vi "Process.vi"(8 "error in":errorcluster, 11 "Logger":refnum<class "Logger.PGSQL.lvclass">) -> (0 "error out":errorcluster, 3 "Logger out":refnum<class "Logger.PGSQL.lvclass">)   [LabVIEW 2019, in "Logger.PGSQL.lvclass"]
doc: "---------------------------------------------------------------\nJKI State Machine Objects™\nhttp://jki.net/state-machine-objects/\nCopyright (C) 2005-2015, JKI <info@jki.net>\nALL RIGHTS RESERVED"
uses:
  Logger.PGSQL.lvclass
  C:/Program Files (x86)/National Instruments/LabVIEW 2019/vi.lib/JKI/JKI SMO/SMO/SMO.lvclass
  C:/Program Files (x86)/National Instruments/LabVIEW 2019/user.lib/LevyLab/Logger/Logger.lvclass
  <userlib>/LevyLab/LV-Data/LV-Data.PG/LV-Data.PGSQL.lvclass
  <vilib>/JKI/JKI SMO/SMO/SMO.lvclass/SMO.ctl
  <vilib>/JKI/JKI SMO/SMO/Private/ReftoDVR--SMO.vi
  <userlib>/LevyLab/LV-Data/LV-Data.PG/API/Write Variable (one-row).vi
  <userlib>/LevyLab/LV-Data/LV-Data.PG/API/Read Variable (string).vi
  <userlib>/LevyLab/Logger/Logger.lvclass
  <vilib>/JKI/JKI SMO/SMO/SMO.lvclass
panel:
  out "State History":string
  out "Status":string
  out "Data":variant
  out "Address(es)":string
  # "DB Logger"
  # "For instructions on how to use the JKI State Machine Objects, examples and video tutorials, visit:\nhttp://jki.net/state-machine-objects/\n\nJKI State Machine Objects™\nhttp://jki.net/state-machine-objects/\nCopyright (C) 2005-2015, JKI <info@jki.net>\nALL RIGHTS RESERVED"
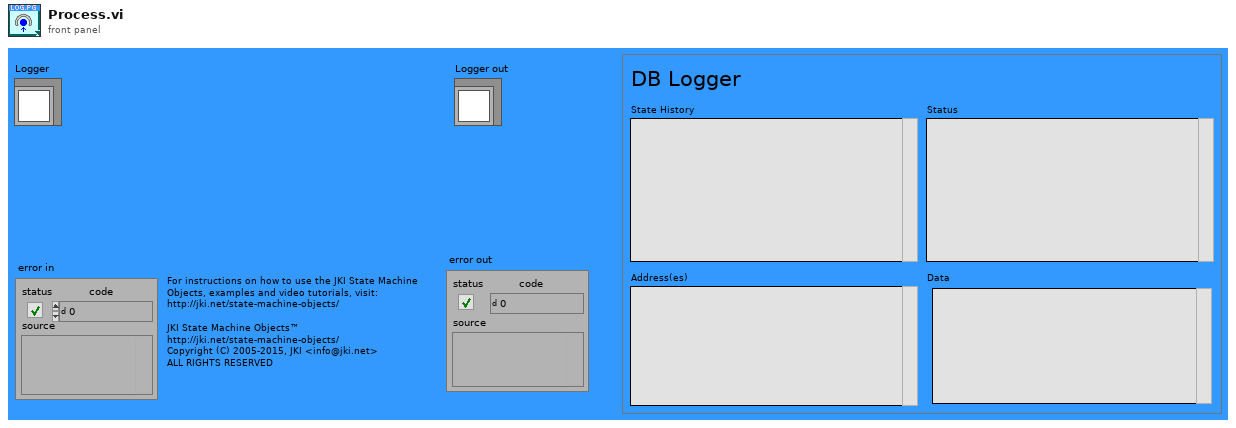
[diagram p1: front panel]
types:
  T1 = enum32{"invalid app kind", "Development System", "Run Time System", "Student Edition", "Embedded LabVIEW", "Evaluation", "Custom"}
  T2 = enum32{"Invalid", "Standard", "Closed", "Hidden", "Minimized", "Maximized"}
  T3 = enum32{"Bad", "Idle", "Run top level", "Running"}
  T4 = cluster{"Core":cluster{"Current VI Reference":refnum<vi>, "Close Panel on Exit?":bool, "Last Error":cluster{"error":errorcluster, "previous state":string, "remaining states":string}, "Shutdown?":bool}, "SelfRef":refnum<class "Logger.PGSQL.lvclass">, "Data.PGSQL":refnum<class "LV-Data.PGSQL.lvclass">, "variable address":string, "data in":variant, "data out":variant, "Debug Mode?":bool, "Time":timestamp}
  T5 = cluster{"Current VI Reference":refnum<vi>, "Close Panel on Exit?":bool, "Last Error":cluster{"error":errorcluster, "previous state":string, "remaining states":string}, "Shutdown?":bool}
  T6 = typedef "SMO.lvclass/Protected Events.ctl" = cluster{"StopProcesses":refnum<user-event>, "AbortProcesses":refnum<user-event>, "Config Changed":refnum<user-event>, "Dependency":refnum<user-event>}
  T7 = typedef "Logger.PGSQL.lvclass/PrivateEvents--Cluster.ctl" = cluster{"Set Address":refnum<user-event>, "Write Variable":refnum<user-event>, "Read Variable":refnum<user-event>}
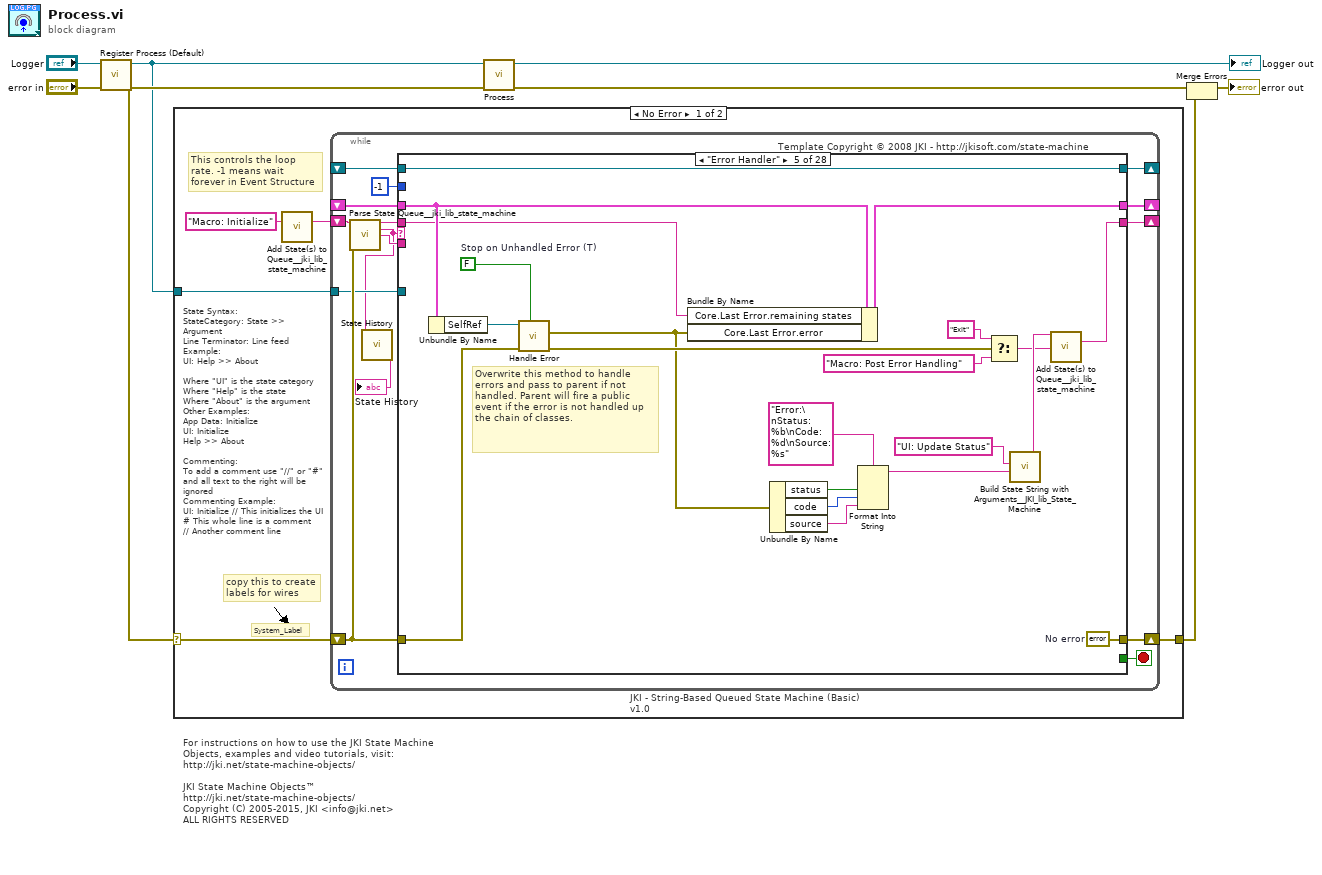
[diagram p0: block diagram]
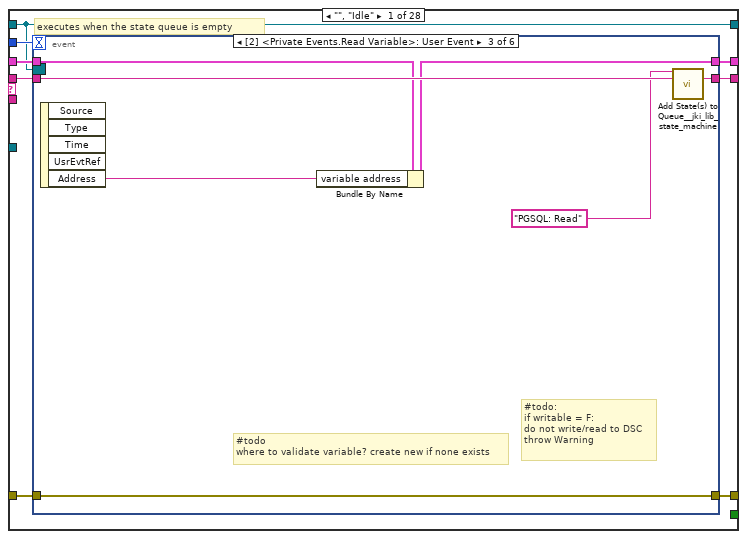
[diagram p2: hidden frame]
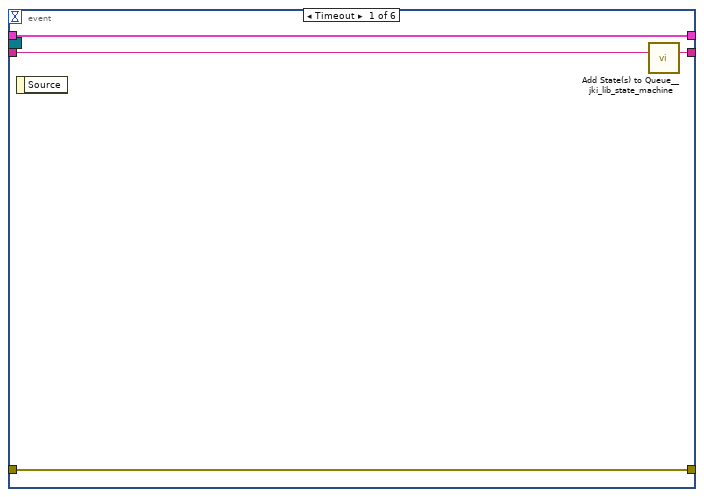
[diagram p3: hidden frame]
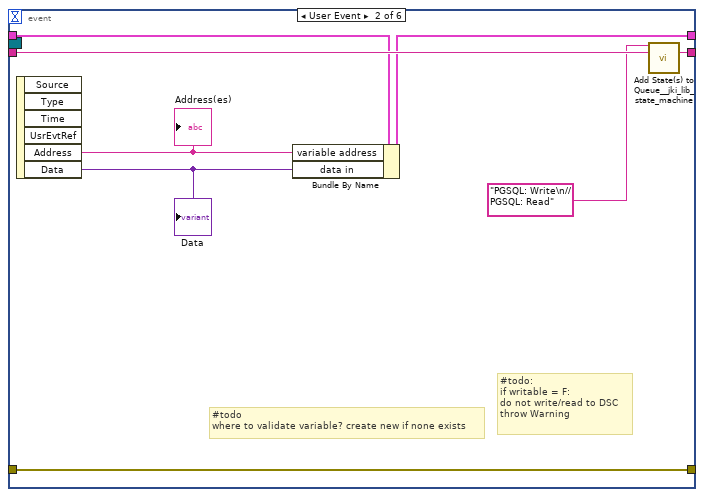
[diagram p4: hidden frame]
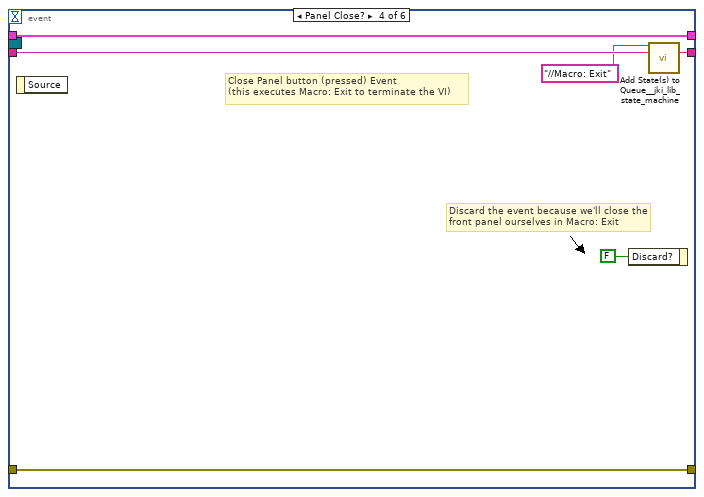
[diagram p5: hidden frame]
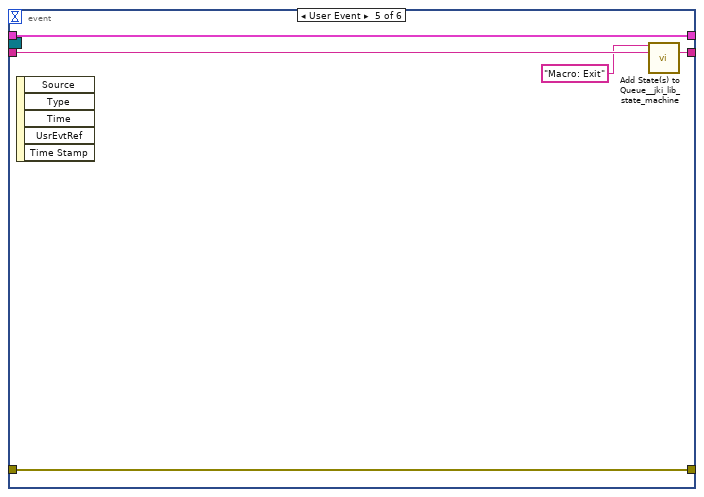
[diagram p6: hidden frame]
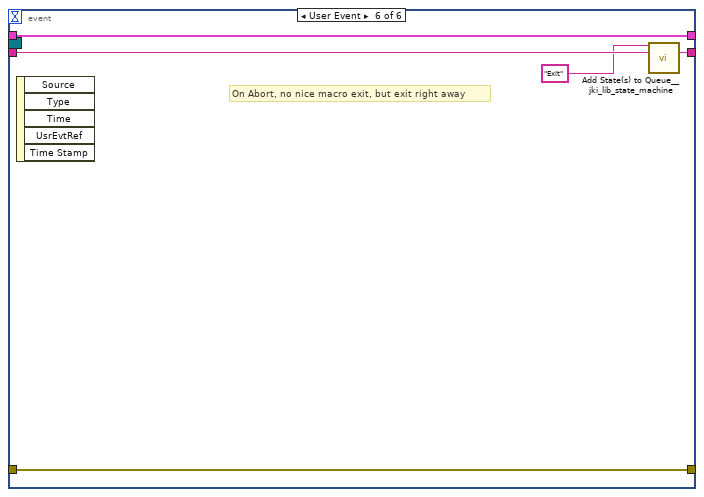
[diagram p7: hidden frame]
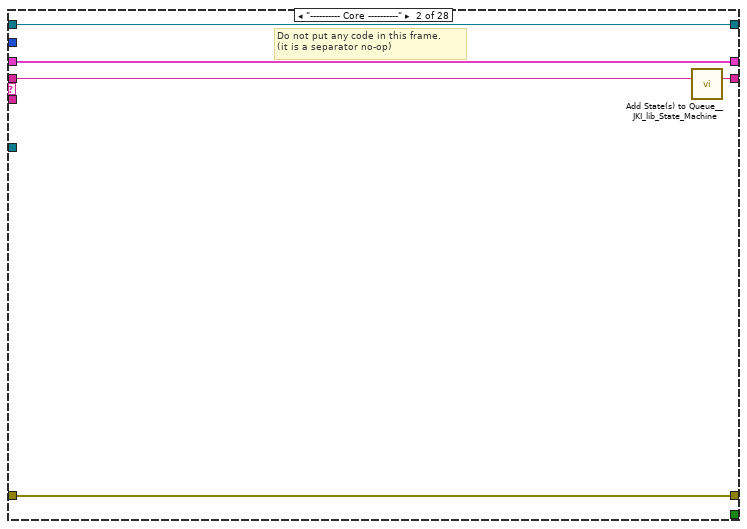
[diagram p8: hidden frame]
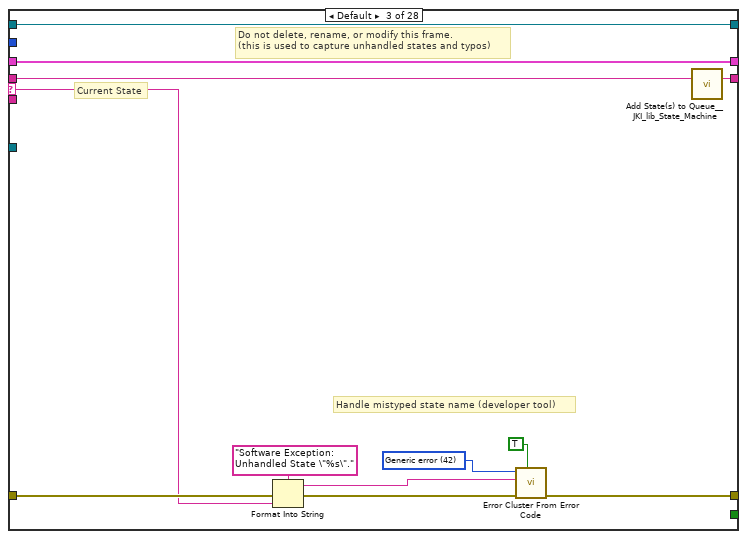
[diagram p9: hidden frame]
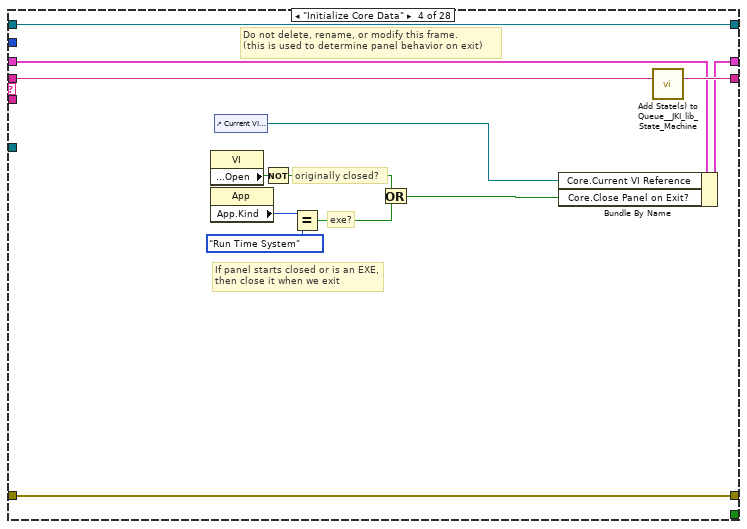
[diagram p10: hidden frame]
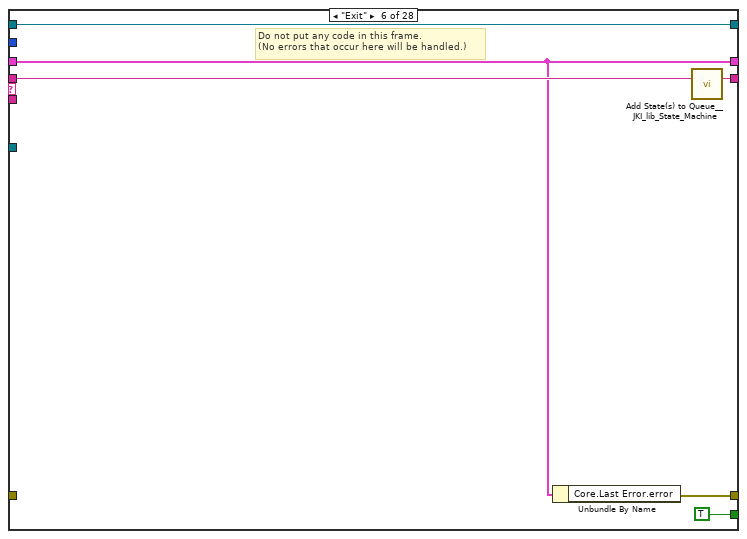
[diagram p11: hidden frame]
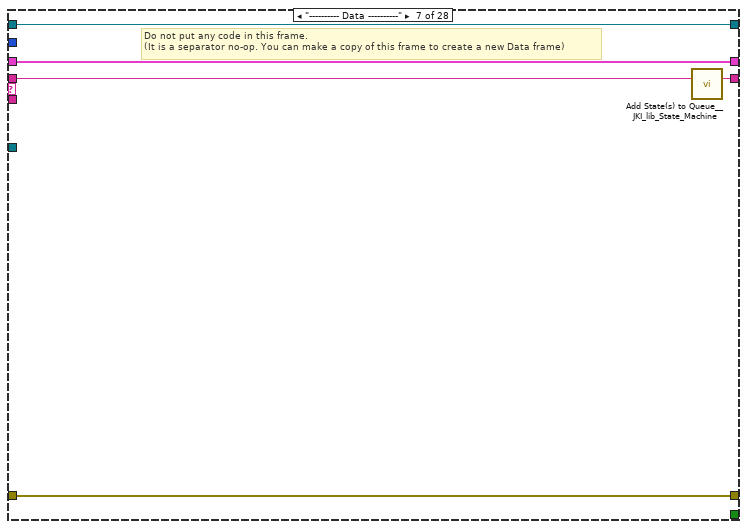
[diagram p12: hidden frame]
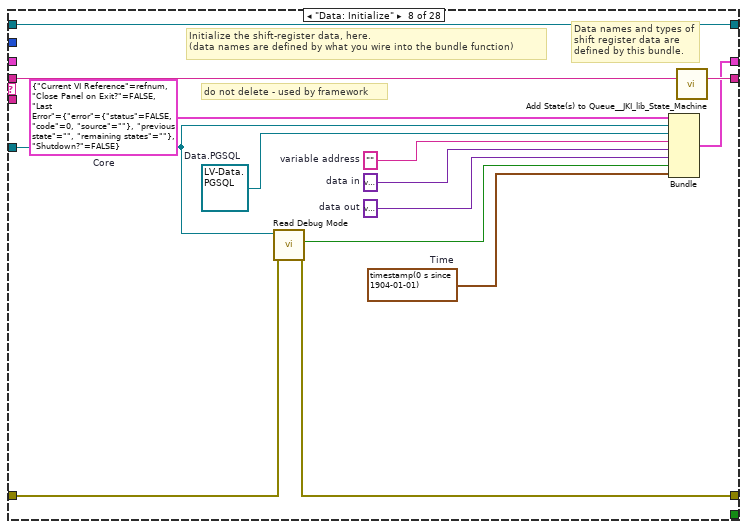
[diagram p13: hidden frame]
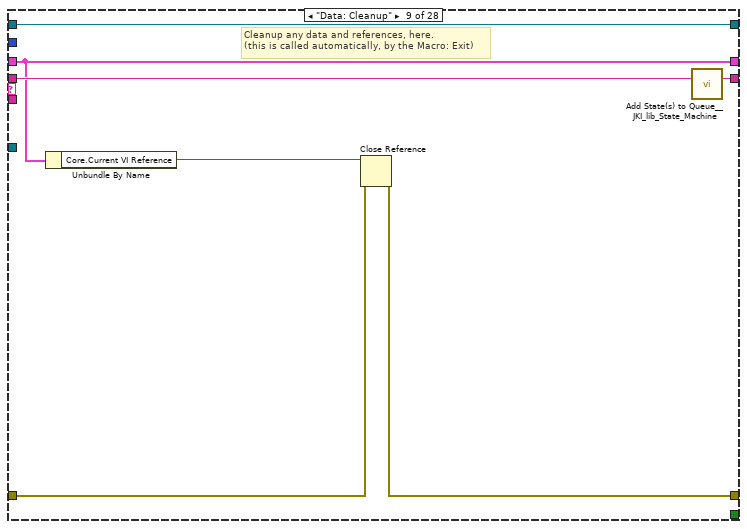
[diagram p14: hidden frame]
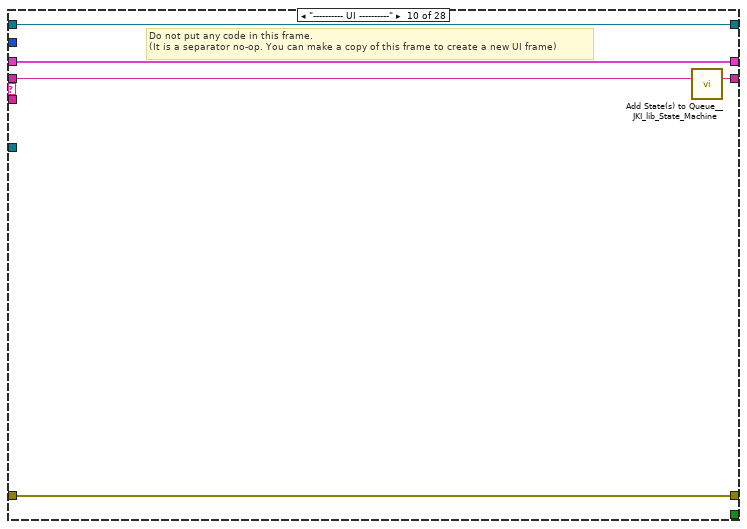
[diagram p15: hidden frame]
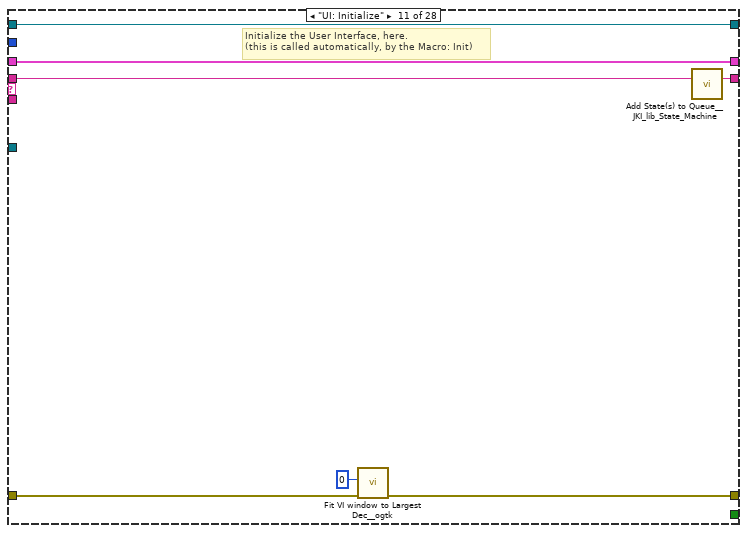
[diagram p16: hidden frame]
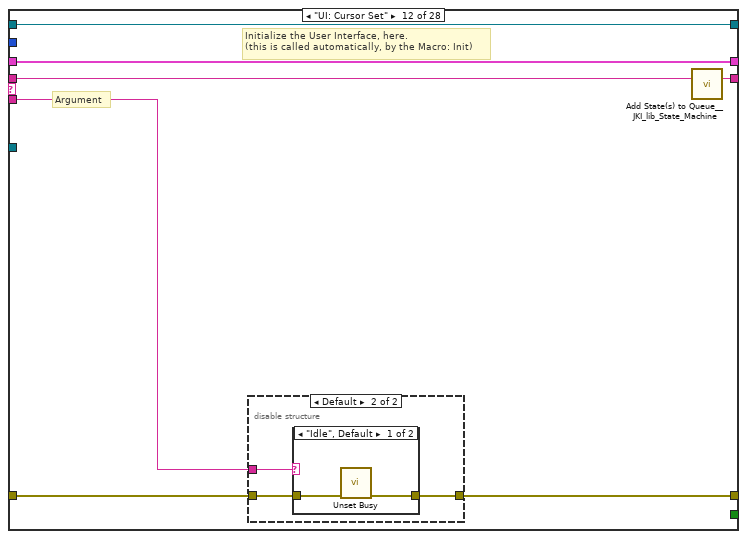
[diagram p17: hidden frame]
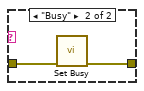
[diagram p19: hidden frame]
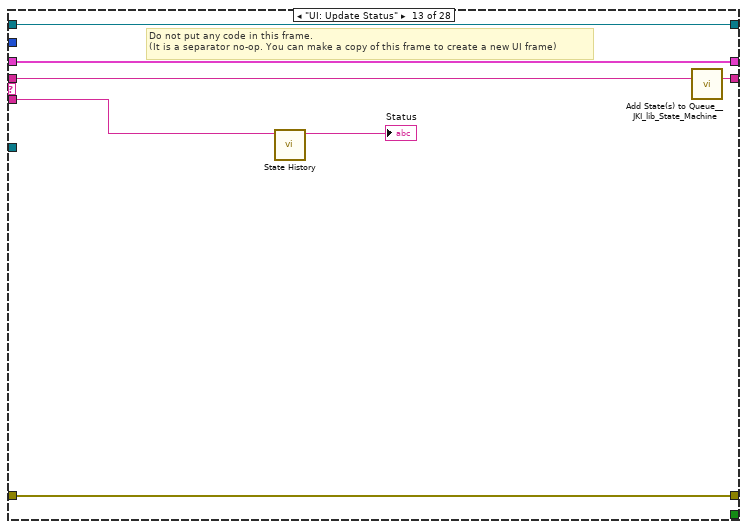
[diagram p20: hidden frame]
diagram:
  # "For instructions on how to use the JKI State Machine Objects, examples and video tutorials, visit:\nhttp://jki.net/state-machine-objects/\n\nJKI State Machine Objects™\nhttp://jki.net/state-machine-objects/\nCopyright (C) 2005-2015, JKI <info@jki.net>\nALL RIGHTS RESERVED"
  n1 = call <vilib>:"Register Process (Default).vi"("error in (no error)"="error in", "SMO"="Logger") -> ("error out"=w5:errorcluster, "SelfRef"=w4:refnum<class "Logger.PGSQL.lvclass">)  [unwired: 8 in]
  n2 = case shown="No Error" w5 {
    selector: w5 -> [w10 w412]
    tunnel: w4 -> [w11 _]
    tunnel: [w9 w412] -> w2
    frame No Error {
      # "State Syntax:\nStateCategory: State >> Argument\nLine Terminator: Line feed\nExample:\nUI: Help >> About\n\nWhere \"UI\" is the state category\nWhere \"Help\" is the state\nWhere \"About\" is the argument\nOther Examples:\nApp Data: Initialize\nUI: Initialize\nHelp >> About\n\nCommenting:\nTo add a comment use \"//\" or \"#\" and all text to the right will be ignored\nCommenting Example:\nUI: Initialize // This initializes the UI\n# This whole line is a comment\n// Another comment line"
      # "copy this to create labels for wires"
      # "This controls the loop rate. -1 means wait forever in Event Structure"
      # "System_Label"
      n3 = call <vilib>:"Add State(s) to Queue__jki_lib_state_machine.vi"("State(s) in (\"\")"="Macro: Initialize") -> ("States Out"=w13:string)  [unwired: 14 in]
      n4 = while "JKI - String-Based Queued State Machine (Basic) v1.0" {
        shift-right: [w22] -> _
        shift-left: _ -> [w21]
        shift-right: [w25] -> w9
        shift-left: w10 -> [w19]
        shift-right: [w24] -> _
        shift-left: w13 -> [w26]
        tunnel: w11 -> [w18]
        shift-right: [w17] -> _
        shift-left: _ -> [w16]
        stop <- w23 stop-if-true
        # "Template Copyright © 2008 JKI - http://jkisoft.com/state-machine"
        n5 = call <vilib>:"Parse State Queue__jki_lib_state_machine.vi"("State Queue"=w26, "Error In (no error)"=w19) -> ("Remaining States"=w28:string, "Current State"=w14:string, "Arguments"=w27:string)  [unwired: 11 in]
        n6 = call <userlib>:"State History.vi"("Current State"=w14) -> ("History"=→"State History":string)  [unwired: 10 in]
        n7 = case shown="\"Error Handler\"" w14 {
          selector: w14 -> [_ _ w78 _ _ _ _ _ _ _ _ _ _ _ _ _ _ _ _ _ _ _ _ _ _ _ _ _]
          tunnel: w28 -> [w36 w76 w82 w101 w108 w128 w133 w147 w154 w159 w166 w173 w188 w196 w228 w251 w263 w286 w291 w302 w307 w320 w326 w331 w340 w364 w394 w411]
          tunnel: w27 -> [_ _ _ _ _ _ _ _ _ _ _ w167 w182 w190 _ _ _ _ _ _ _ _ _ _ _ _ _ _]
          tunnel: w21 -> [w34 w73 w80 w92 w118 w124 w130 _ w149 w156 w164 w171 w185 w192 w225 w236 w253 w278 w288 w299 w304 w318 w324 w329 w332 w359 w387 w406]
          tunnel: [w33 w74 w84 w98 w119 w123 w131 w140 w150 w157 w162 w168 w186 w193 w226 w232 w261 w284 w289 w293 w305 w313 w322 w327 w335 w361 w391 w403] -> w25
          tunnel: w19 -> [w32 w74 w83 w98 w120 _ w131 w134 w151 w157 w161 w169 w186 w194 w226 w231 w261 w284 w289 w294 w305 w314 w322 w327 w333 w356 w388 w404]
          tunnel: [w35 w75 w81 w100 w104 w127 w132 w146 w153 w158 w165 w172 w187 w195 w227 w250 w262 w285 w290 w301 w306 w319 w325 w330 w339 w363 w393 w410] -> w24
          tunnel: [_ _ _ _ _ TRUE _ _ _ _ _ _ _ _ _ _ _ _ _ _ _ _ _ _ _ _ _ _] -> w23
          tunnel: [w31 w73 w80 w99 w117 w124 w130 w145 w149 w156 w164 w171 w185 w192 w225 w236 w254 w278 w288 w299 w304 w318 w324 w329 w337 w358 w387 w405] -> w22
          tunnel: -1 ("Timeout") -> [w30 _ _ _ _ _ _ _ _ _ _ _ _ _ _ _ _ _ _ _ _ _ _ _ _ _ _ _]
          tunnel: w18 -> [_ _ _ _ _ _ _ w135 _ _ _ _ _ _ _ w230 _ _ _ _ _ _ _ _ _ _ _ _]
          tunnel: [w29 w72 w77 w89 w122 w125 w129 w144 w148 w155 w163 w170 w184 w189 w224 w249 w260 w279 w287 w300 w303 w317 w323 w328 w338 w362 w392 w409] -> w17
          tunnel: w16 -> [w29 w72 w77 w89 w122 w125 w129 w144 w148 w155 w163 w170 w184 w189 w224 w249 w260 w279 w287 w300 w303 _ w323 w328 w338 w362 w392 w409]
          frame "", "Idle" {
            # "executes when the state queue is empty"
            n8 = event shown="[2] <Private Events.Read Variable>: User Event" {
              selector: w29 -> [_ _ _ _ _ _]
              dyn-events: _ -> [_ _ _ _ _ _]
              timeout: w30 -> [_ _ _ _ _ _]
              tunnel: w36 -> [w40 w48 w55 w61 w66 w71]
              tunnel: [w39 w47 w54 w60 w65 w70] -> w35
              tunnel: w34 -> [w38 w45 w52 w58 w63 w68]
              tunnel: [w37 w46 w53 w59 w64 w69] -> w33
              tunnel: w32 -> [w37 w46 w53 w59 w64 w69]
              tunnel: [w38 w44 w51 w58 w63 w68] -> w31
              event Timeout {
                n9 = event-data() -> ()  [unwired: 1 in, 1 out]
                n10 = call <vilib>:"Add State(s) to Queue__jki_lib_state_machine.vi"("State(s) in (\"\")"=w40) -> ("States Out"=w39:string)  [unwired: 14 in]
              }
              event User Event {
                # "#todo:\nif writable = F:\ndo not write/read to DSC\nthrow Warning"
                # "#todo\nwhere to validate variable? create new if none exists"
                n11 = event-data() -> ("Address"=w41:string, "Data"=w42:variant)  [unwired: 1 in, 4 out]
                "Address(es)" <- w41
                "Data" <- w42
                n12 = Bundle By Name(cluster=w45, "variable address"=w41, "data in"=w42) -> (w44:T4)
                n13 = call <vilib>:"Add State(s) to Queue__jki_lib_state_machine.vi"("State(s) in Front (\"\")"="PGSQL: Write\n//PGSQL: Read" ("State(s) in Front (\"\")"), "State(s) in (\"\")"=w48) -> ("States Out"=w47:string)  [unwired: 13 in]
              }
              event User Event {
                # "#todo:\nif writable = F:\ndo not write/read to DSC\nthrow Warning"
                # "#todo\nwhere to validate variable? create new if none exists"
                n14 = event-data() -> ("Address"=w49:string)  [unwired: 1 in, 4 out]
                n15 = Bundle By Name(cluster=w52, "variable address"=w49) -> (w51:T4)
                n16 = call <vilib>:"Add State(s) to Queue__jki_lib_state_machine.vi"("State(s) in Front (\"\")"="PGSQL: Read" ("State(s) in Front (\"\")"), "State(s) in (\"\")"=w55) -> ("States Out"=w54:string)  [unwired: 13 in]
              }
              event Panel Close? {
                # "Discard the event because we'll close the front panel ourselves in Macro: Exit"
                # "Close Panel button (pressed) Event\n(this executes Macro: Exit to terminate the VI)"
                n17 = event-data() -> ()  [unwired: 1 in, 1 out]
                n18 = event-data("Discard?"=FALSE) -> ()  [unwired: 1 in, 1 out]
                n19 = call <vilib>:"Add State(s) to Queue__jki_lib_state_machine.vi"("State(s) in Front (\"\")"="//Macro: Exit", "State(s) in (\"\")"=w61) -> ("States Out"=w60:string)  [unwired: 13 in]
              }
              event User Event {
                n20 = event-data() -> ()  [unwired: 1 in, 5 out]
                n21 = call <vilib>:"Add State(s) to Queue__jki_lib_state_machine.vi"("State(s) in Front (\"\")"="Macro: Exit", "State(s) in (\"\")"=w66) -> ("States Out"=w65:string)  [unwired: 13 in]
              }
              event User Event {
                # "On Abort, no nice macro exit, but exit right away"
                n22 = event-data() -> ()  [unwired: 1 in, 5 out]
                n23 = call <vilib>:"Add State(s) to Queue__jki_lib_state_machine.vi"("State(s) in Front (\"\")"="Exit", "State(s) in (\"\")"=w71) -> ("States Out"=w70:string)  [unwired: 13 in]
              }
            }
          }
          frame "---------- Core ----------" {
            # "Do not put any code in this frame.\n(it is a separator no-op)"
            n24 = call <vilib>:"Add State(s) to Queue__JKI_lib_State_Machine.vi"("State(s) in (\"\")"=w76) -> ("States Out"=w75:string)  [unwired: 14 in]
          }
          frame Default {
            w87 = 42 items=["No error", "Argument error", "Memory is full", "Out of zone", "End of file", "File already open", "Generic file I/O error", "File not found", "File permission error", "Disk is full", "Duplicate path", "Too many files open", "System feature not enabled", "Resource file not found", "Cannot add resource", "Resource not found", "Image not found", "Image memory error", "Pen does not exist", "Config type invalid", "Config token not found", "Config parse error", "Config memory error", "Bad external code format", "Bad external code offset", "External code not present", "Null window", "Destroy window error", "Null menu", "Print aborted", "Bad print record", "Print driver error", "Windows error during printing", "Memory error during printing", "Print dialog error", "Generic print error", "Invalid device refnum", "Device not found", "Device parameter error", "Device unit error", "Cannot open device", "Device call aborted", "Generic error", "Cancelled by user", "Object ID too low", "Object ID too high", "Object not in heap", "Unknown heap", "Unknown object (invalid DefProc)", "Unknown object (DefProc not in table)", "Message out of range", "Invalid (null) method", "Unknown message", "Manager call not supported", "Bad address", "Network operation in progress", "Network operation timed out", "Connection is busy", "Network attribute not supported", "Network error", "Address in use", "System out of memory", "Connection aborted", "Connection refused", "Not connected", "Already connected", "Connection closed", "Initialization error (interapplication manager)", "Bad occurrence", "Wait on unbound occurrence handler", "Occurrence queue overflow", "Datalog type conflict", "Unused", "Unrecognized type (interapplication manager)", "Memory corrupt", "Failed to make temporary DLL", "Old CIN version", "Drag socket not found", "Failed to load drop-object", "Failed to register OLE object", "Failed to release OLE object", "Format specifier type mismatch", "Unknown format specifier", "Too few format specifiers", "Too many format specifiers", "Scan failed", "Newer CIN version", "Error converting to variant", "Runtime menu error", "Password tampered", "Variant attribute not found", "Incompatible variant data type", "Event data is not available", "Event Store is not present", "Occurrence is not found", "Event Queue is not created", "Event info is not available", "Refnum passed is NULL", "Error retrieving Class GUID", "Error retrieving CoClass GUID", "Error retrieving TypeLib GUID.", "Bad built application magic bytes.", "Specific driver is different from the specific driver associated with the Logical Name.", "There is no session opened to the class driver.", "Max Error", "MAX - Error with config objects", "MAX - Error loading configuration", "MAX - Group not supported"]
            # "Current State"
            # "Do not delete, rename, or modify this frame.\n(this is used to capture unhandled states and typos)"
            # "Handle mistyped state name (developer tool)"
            n25 = Format Into String(format string="Software Exception: Unhandled State \"%s\"." ("message"), error in=w83, w78) -> (resulting string=w86:string, error out=w85:errorcluster)  [unwired: 1 in]
            n26 = call <vilib>:"Error Cluster From Error Code.vi"("show call chain? (False)"=TRUE, "error in (no error)"=w85, "error message (\"\")"=w86, "error code (0)"=w87) -> ("error out"=w84:errorcluster)  [unwired: 5 in]
            n27 = call <vilib>:"Add State(s) to Queue__JKI_lib_State_Machine.vi"("State(s) in (\"\")"=w82) -> ("States Out"=w81:string)  [unwired: 14 in]
          }
          frame "Initialize Core Data" {
            # "Do not delete, rename, or modify this frame.\n(this is used to determine panel behavior on exit)"
            # "originally closed?"
            # "exe?"
            # "If panel starts closed or is an EXE, then close it when we exit"
            n28 = property class="VI"() -> ("Front Panel.Open"=w97:bool)  [unwired: 2 in, 2 out]
            n29 = property class="App"() -> ("App.Kind"=w96:T1)  [unwired: 2 in, 2 out]
            n30 = control-ref of="Current VI Reference"() -> (w90:refnum<vi>)
            n31 = Not(x=w97) -> (.not. x?=w94:bool)
            n32 = Equal?(x=w96, y=T1."Run Time System" ("Application:Kind")) -> (x = y?=w93:bool)
            n33 = Or(x=w94, y=w93) -> (x .or. y?=w91:bool)
            n34 = Bundle By Name(cluster=w92, "Core.Current VI Reference"=w90, "Core.Close Panel on Exit?"=w91) -> (w99:T4)
            n35 = call <vilib>:"Add State(s) to Queue__JKI_lib_State_Machine.vi"("State(s) in (\"\")"=w101) -> ("States Out"=w100:string)  [unwired: 14 in]
          }
          frame "Error Handler" {
            w114 = FALSE  # Stop on Unhandled Error (T)
            w119 = errorcluster {"status"=FALSE, "code"=0, "source"=""}  # No error
            # "Overwrite this method to handle errors and pass to parent if not handled. Parent will fire a public event if the error is not handled up the chain of classes."
            n36 = Unbundle By Name(w118) -> ("SelfRef"=w121:refnum<class "Logger.PGSQL.lvclass">)
            n37 = call-dynamic "Handle Error.vi"("Stop on Unhandled Error (T)"=w114, "error in"=w120, "SMO"=w121) -> ("handling error"=w115:errorcluster, "Unhandled error"=w113:errorcluster)  [unwired: 6 in, 1 out]
            n38 = Bundle By Name(cluster=w118, "Core.Last Error.remaining states"=w108, "Core.Last Error.error"=w113) -> (w117:T4)
            n39 = Unbundle By Name(w113) -> ("status"=w112:bool, "code"=w110:i32, "source"=w109:string)
            n40 = Format Into String(format string="Error:\nStatus: %b\nCode: %d\nSource: %s", w112, w110, w109) -> (resulting string=w103:string)  [unwired: 2 in, 1 out]
            n41 = Select(t="Exit", s=w115, f="Macro: Post Error Handling") -> (s? t:f=w105:string)
            n42 = call <vilib>:"Build State String with Arguments__JKI_lib_State_Machine.vi"("Arguments (\"\")"=w103, "State"="UI: Update Status") -> ("State with Arguments"=w106:string)  [unwired: 4 in]
            n43 = call <vilib>:"Add State(s) to Queue__jki_lib_state_machine.vi"("State(s) in Front (\"\")"=w106, "State(s) at Back (\"\")"=w105) -> ("States Out"=w104:string)  [unwired: 13 in]
          }
          frame "Exit" {
            # "Do not put any code in this frame.\n(No errors that occur here will be handled.)"
            n44 = Unbundle By Name(w124) -> ("Core.Last Error.error"=w123:errorcluster)
            n45 = call <vilib>:"Add State(s) to Queue__JKI_lib_State_Machine.vi"("State(s) in (\"\")"=w128) -> ("States Out"=w127:string)  [unwired: 14 in]
          }
          frame "---------- Data ----------" {
            # "Do not put any code in this frame.\n(It is a separator no-op. You can make a copy of this frame to create a new Data frame)"
            n46 = call <vilib>:"Add State(s) to Queue__JKI_lib_State_Machine.vi"("State(s) in (\"\")"=w133) -> ("States Out"=w132:string)  [unwired: 14 in]
          }
          frame "Data: Initialize" {
            w136 = timestamp(0 s since 1904-01-01)  # Time
            w137 = refnum<class "LV-Data.PGSQL.lvclass"> refnum  # Data.PGSQL
            w138 = variant  # data out
            w141 = variant  # data in
            w142 = ""  # variable address
            w143 = T5 {"Current VI Reference"=refnum, "Close Panel on Exit?"=FALSE, "Last Error"={"error"={"status"=FALSE, "code"=0, "source"=""}, "previous state"="", "remaining states"=""}, "Shutdown?"=FALSE}  # Core
            # "do not delete - used by framework"
            # "Data names and types of shift register data are defined by this bundle."
            # "Initialize the shift-register data, here.\n(data names are defined by what you wire into the bundle function)"
            n47 = call <userlib>:"Read Debug Mode.vi"("error in (no error)"=w134, "Logger in"=w135) -> ("error out"=w140:errorcluster, "Debug Mode?"=w139:bool)  [unwired: 7 in, 1 out]
            n48 = Bundle("Core"=w143, "SelfRef"=w135, "Data.PGSQL"=w137, "variable address"=w142, "data in"=w141, "data out"=w138, "Debug Mode?"=w139, "Time"=w136) -> (w145:T4)  [unwired: 1 in]
            n49 = call <vilib>:"Add State(s) to Queue__JKI_lib_State_Machine.vi"("State(s) in (\"\")"=w147) -> ("States Out"=w146:string)  [unwired: 14 in]
          }
          frame "Data: Cleanup" {
            # "Cleanup any data and references, here.\n(this is called automatically, by the Macro: Exit)"
            n50 = Unbundle By Name(w149) -> ("Core.Current VI Reference"=w152:refnum<vi>)
            n51 = Close Reference(reference=w152, error in (no error)=w151) -> (error out=w150:errorcluster)
            n52 = call <vilib>:"Add State(s) to Queue__JKI_lib_State_Machine.vi"("State(s) in (\"\")"=w154) -> ("States Out"=w153:string)  [unwired: 14 in]
          }
          frame "---------- UI ----------" {
            # "Do not put any code in this frame.\n(It is a separator no-op. You can make a copy of this frame to create a new UI frame)"
            n53 = call <vilib>:"Add State(s) to Queue__JKI_lib_State_Machine.vi"("State(s) in (\"\")"=w159) -> ("States Out"=w158:string)  [unwired: 14 in]
          }
          frame "UI: Initialize" {
            # "Initialize the User Interface, here.\n(this is called automatically, by the Macro: Init)"
            n54 = call <userlib>:"Fit VI window to Largest Dec__ogtk.vi"("error in (no error)"=w161, "border spacing (2 px)"=0) -> ("error out"=w162:errorcluster)  [unwired: 4 in, 1 out]
            n55 = call <vilib>:"Add State(s) to Queue__JKI_lib_State_Machine.vi"("State(s) in (\"\")"=w166) -> ("States Out"=w165:string)  [unwired: 14 in]
          }
          frame "UI: Cursor Set" {
            # "Argument"
            # "Initialize the User Interface, here.\n(this is called automatically, by the Macro: Init)"
            n56 = disable-structure shown="Default" {
              disable-tunnel: w169 -> [w174 w177]
              disable-tunnel: [w174 w176] -> w168
              disable-tunnel: w167 -> [_ w175]
              frame condition #0 {
              }
              frame condition #1 (active) {
                n57 = case shown="\"Idle\", Default" w175 {
                  tunnel: w177 -> [w179 w181]
                  tunnel: [w178 w180] -> w176
                  frame "Idle", Default {
                    n58 = call <vilib>:"Unset Busy.vi"("error in (no error)"=w179) -> ("error out"=w178:errorcluster)  [unwired: 10 in]
                  }
                  frame "Busy" {
                    n59 = call <vilib>:"Set Busy.vi"("error in (no error)"=w181) -> ("error out"=w180:errorcluster)  [unwired: 9 in, 1 out]
                  }
                }
              }
            }
            n60 = call <vilib>:"Add State(s) to Queue__JKI_lib_State_Machine.vi"("State(s) in (\"\")"=w173) -> ("States Out"=w172:string)  [unwired: 14 in]
          }
          frame "UI: Update Status" {
            # "Do not put any code in this frame.\n(It is a separator no-op. You can make a copy of this frame to create a new UI frame)"
            n61 = call <userlib>:"State History.vi"("Current State"=w182) -> ("History"=→"Status":string)  [unwired: 10 in]
            n62 = call <vilib>:"Add State(s) to Queue__JKI_lib_State_Machine.vi"("State(s) in (\"\")"=w188) -> ("States Out"=w187:string)  [unwired: 14 in]
          }
          frame "UI: Front Panel State" {
            # "Argument"
            # "Set Front Panel Open or Closed\n(Usage: \"UI: Front Panel State >> Open|Close\")"
            n63 = Unbundle By Name(w192) -> ("Core.Current VI Reference"=w191:refnum<vi>)
            n64 = disable-structure shown="Default" {
              disable-tunnel: w194 -> [w200 w223]
              disable-tunnel: [w199 w223] -> w193
              disable-tunnel: w191 -> [w198 _]
              disable-tunnel: w190 -> [w197 _]
              frame condition #0 (active) {
                n65 = case shown="\"Close\"" w197 {
                  tunnel: w200 -> [w204 w217]
                  tunnel: [w206 w218] -> w199
                  tunnel: w198 -> [w205 w215]
                  frame "Open", Default {
                    n66 = property class="VI"(reference=w205, error in=w204) -> (reference out=w202:refnum<vi>, error out=w203:errorcluster, "FP.State"=w201:T2)
                    n67 = case shown="\"Closed\"" w201 {
                      tunnel: [w209 w212] -> w206
                      tunnel: w203 -> [w208 w212]
                      tunnel: w202 -> [w207 _]
                      frame "Closed" {
                        n68 = invoke class="VI" method="FP.Open"(reference=w207, error in=w208, "Activate"=TRUE, "State"=T2."Standard") -> (error out=w209:errorcluster)  [unwired: 1 in, 4 out]
                      }
                      frame Default {
                      }
                    }
                  }
                  frame "Close" {
                    n69 = property class="VI"(reference=w215, error in=w217) -> (reference out=w214:refnum<vi>, error out=w216:errorcluster, "FP.State"=w213:T2)
                    n70 = case shown="Default" w213 {
                      tunnel: [w219 w222] -> w218
                      tunnel: w216 -> [w219 w221]
                      tunnel: w214 -> [_ w220]
                      frame "Invalid", "Closed" {
                      }
                      frame Default {
                        n71 = invoke class="VI" method="FP.Close"(reference=w220, error in=w221) -> (error out=w222:errorcluster)  [unwired: 1 in, 2 out]
                      }
                    }
                  }
                }
              }
              frame condition #1 {
              }
            }
            n72 = call <vilib>:"Add State(s) to Queue__JKI_lib_State_Machine.vi"("State(s) in (\"\")"=w196) -> ("States Out"=w195:string)  [unwired: 14 in]
          }
          frame "---------- Macro ----------" {
            # "Do not put any code in this frame.\n(It is a separator no-op. You can make a copy of this frame to create a new Macro frame)"
            n73 = call <vilib>:"Add State(s) to Queue__JKI_lib_State_Machine.vi"("State(s) in (\"\")"=w228) -> ("States Out"=w227:string)  [unwired: 14 in]
          }
          frame "Macro: Initialize" {
            w241 = "Process: Sync"
            # "This needs to be called here before Data: Initialize\nto ensure that the correct argument is present"
            # "Initialization Macro\n(This is called once, when the VI starts)"
            n74 = control-ref of="This VI"() -> (w243:refnum<vi>)
            n75 = property class="VI"(reference=w243) -> ("Exec.State"=w242:T3)  [unwired: 1 in, 2 out]
            n76 = call <userlib>:"Read Debug Mode.vi"("error in (no error)"=w231, "Logger in"=w230) -> ("error out"=w232:errorcluster, "Debug Mode?"=w229:bool)  [unwired: 7 in, 1 out]
            n77 = Equal?(x=w242, y=T3."Run top level") -> (x = y?=w247:bool)
            n78 = Select(t="Open", s=w229, f="Close") -> (s? t:f=w238:string)
            n79 = Select(t=w241, s=w247, f="") -> ()  [unwired: 1 out]
            n80 = call <vilib>:"Build State String with Arguments__JKI_lib_State_Machine.vi"("Arguments (\"\")"=w238, "State"="UI: Front Panel State") -> ("State with Arguments"=w235:string)  [unwired: 4 in]
            n81 = call <vilib>:"Add State(s) to Queue__JKI_lib_State_Machine.vi"("State(s) in Front (\"\")"="UI: Initialize", "State(s) in (\"\")"=w235) -> ("States Out"=w233:string)  [unwired: 13 in]
            n82 = call <vilib>:"Add State(s) to Queue__JKI_lib_State_Machine.vi"("State(s) in Front (\"\")"="Data: Initialize\nInitialize Core Data\nEvents: Register\nPGSQL: Open", "State(s) in (\"\")"=w241, "State(s) at Back (\"\")"=w233) -> ("States Out"=w244:string)  [unwired: 12 in]
            n83 = call <vilib>:"Add State(s) to Queue__JKI_lib_State_Machine.vi"("State(s) in Front (\"\")"=w244, "State(s) in (\"\")"=w251) -> ("States Out"=w250:string)  [unwired: 13 in]
          }
          frame "Macro: Post Error Handling" {
            # "Clear Last Error?"
            n84 = Unbundle By Name(w253) -> ("Core.Last Error.remaining states"=w255:string, "Core.Shutdown?"=w256:bool)
            n85 = Unbundle By Name(w253) -> ("Core.Last Error.error"=w259:errorcluster)
            n86 = case shown="False" FALSE {
              tunnel: w259 -> [w267 _]
              tunnel: [w267 _] -> w258
              frame False {
              }
              frame True {
              }
            }
            n87 = case shown="True" w256 {
              tunnel: w255 -> [w264 w266]
              tunnel: [w264 w265] -> w252
              frame False {
                # "These are the remaining states (at the moment the error occured). States can be altered according to business logic."
                # "NOT SHUTTING DOWN"
              }
              frame True {
                # "Developer can decide to alter the states but should be aware that during the shutdown process, there are certain states that must be run for the SMO to properly shut itself (and this process) down. As such, one can add states to perform additional clean-ups, but should append the remaining state to be executed."
                # "SHUTTING DOWN"
                n88 = call <vilib>:"Add State(s) to Queue__jki_lib_state_machine.vi"("State(s) in (\"\")"=w266) -> ("States Out"=w265:string)  [unwired: 14 in]
              }
            }
            n89 = Bundle By Name(cluster=w253, "Core.Last Error.error"=w258) -> (w254:T4)
            n90 = call <vilib>:"Add State(s) to Queue__JKI_lib_State_Machine.vi"("State(s) in Front (\"\")"=w252, "State(s) in (\"\")"=w263) -> ("States Out"=w262:string)  [unwired: 13 in]
          }
          frame "Macro: Exit" {
            # "Exit Macro\n(This is called once, when the VI exits)"
            n91 = Unbundle By Name(w278) -> ("Debug Mode?"=w269:bool, "Core.Close Panel on Exit?"=w283:bool)
            n92 = Select(t="Open", s=w269, f="Close") -> (s? t:f=w271:string)
            n93 = call <vilib>:"Build State String with Arguments__JKI_lib_State_Machine.vi"("Arguments (\"\")"=w271, "State"="UI: Front Panel State") -> ("State with Arguments"=w268:string)  [unwired: 4 in]
            n94 = Select(t=w268, s=w283, f="") -> (s? t:f=w281:string)
            n95 = call <vilib>:"Add State(s) to Queue__JKI_lib_State_Machine.vi"("State(s) in Front (\"\")"="PGSQL: Close\nData: Cleanup\nEvents: Unregister", "State(s) in (\"\")"="Process: Sync", "State(s) at Back (\"\")"="Exit") -> ("States Out"=w275:string)  [unwired: 12 in]
            n96 = call <vilib>:"Add State(s) to Queue__JKI_lib_State_Machine.vi"("State(s) in (\"\")"=w281, "State(s) at Back (\"\")"=w275) -> ("States Out"=w280:string)  [unwired: 13 in]
            n97 = call <vilib>:"Add State(s) to Queue__JKI_lib_State_Machine.vi"("State(s) in Front (\"\")"=w280, "State(s) in (\"\")"=w286) -> ("States Out"=w285:string)  [unwired: 13 in]
          }
          frame "---------- Process ----------" {
            # "Template Separator\n(You can make a copy of, or modify, this frame)"
            n98 = call <vilib>:"Add State(s) to Queue__JKI_lib_State_Machine.vi"("State(s) in (\"\")"=w291) -> ("States Out"=w290:string)  [unwired: 14 in]
          }
          frame "Process: Sync" {
            n99 = Unbundle By Name(w299) -> ("SelfRef"=w295:refnum<class "Logger.PGSQL.lvclass">)
            n100 = call <vilib>:"WaitOnProcessSync.vi"("error in (no error)"=w294, "SMO"=w295) -> ("error out"=w293:errorcluster, "Don't run?"=w298:bool)  [unwired: 7 in, 1 out]
            n101 = Select(t="Data: Cleanup\nEvents: Unregister\nExit", s=w298, f="") -> (s? t:f=w292:string)
            n102 = call <vilib>:"Add State(s) to Queue__JKI_lib_State_Machine.vi"("State(s) in Front (\"\")"=w292, "State(s) in (\"\")"=w302) -> ("States Out"=w301:string)  [unwired: 13 in]
          }
          frame "---------- Events ----------" {
            # "Template Separator\n(You can make a copy of, or modify, this frame)"
            n103 = call <vilib>:"Add State(s) to Queue__JKI_lib_State_Machine.vi"("State(s) in (\"\")"=w307) -> ("States Out"=w306:string)  [unwired: 14 in]
          }
          frame "Events: Register" {
            # "Expand to add\nmore events"
            n104 = Unbundle By Name(w318) -> ("SelfRef"=w315:refnum<class "Logger.PGSQL.lvclass">)
            n105 = call <vilib>:"GetProtectedEvents.vi"("SMO"=w315) -> ("error out"=w311:errorcluster, "SMO Protected Events"=w316:T6, "SMO out"=w310:refnum<class "Logger.PGSQL.lvclass">)  [unwired: 8 in]
            n106 = call "Logger.GetPrivateEvents.vi"("Logger"=w310) -> ("error out"=w308:errorcluster, "Private Events"=w309:T7)  [unwired: 8 in, 1 out]
            n107 = register-events(w316, w309) -> (reference out=w317:refnum<event-registration>, error out=w312:errorcluster)  [unwired: 2 in]
            n108 = Merge Errors(w308, w314, w312, w311) -> (w313:errorcluster)
            n109 = call <vilib>:"Add State(s) to Queue__JKI_lib_State_Machine.vi"("State(s) in (\"\")"=w320) -> ("States Out"=w319:string)  [unwired: 14 in]
          }
          frame "Events: Unregister" {
            n110 = Unregister For Events(event registration refnum=w323, error in=w322) -> (error out=w321:errorcluster)
            n111 = call <vilib>:"Clear Errors.vi"("error in (no error)"=w321) -> ()  [unwired: 5 in, 2 out]
            n112 = call <vilib>:"Add State(s) to Queue__JKI_lib_State_Machine.vi"("State(s) in (\"\")"=w326) -> ("States Out"=w325:string)  [unwired: 14 in]
          }
          frame "---------- PGSQL ----------" {
            n113 = call <vilib>:"Add State(s) to Queue__JKI_lib_State_Machine.vi"("State(s) in (\"\")"=w331) -> ("States Out"=w330:string)  [unwired: 14 in]
          }
          frame "PGSQL: Open" {
            n114 = Unbundle By Name(w332) -> ("Data.PGSQL"=w334:refnum<class "LV-Data.PGSQL.lvclass">)
            n115 = call <userlib>:"PGSQL.Open.vi"("error in (no error)"=w333, "Data.PG in"=w334) -> ("error out"=w335:errorcluster, "Data.PG out"=w336:refnum<class "LV-Data.PGSQL.lvclass">)  [unwired: 8 in]
            n116 = Bundle By Name(cluster=w332, "Data.PGSQL"=w336) -> (w337:T4)
            n117 = call <vilib>:"Add State(s) to Queue__JKI_lib_State_Machine.vi"("State(s) in (\"\")"=w340) -> ("States Out"=w339:string)  [unwired: 14 in]
          }
          frame "PGSQL: Write" {
            n118 = Unbundle By Name(w359) -> ("Data.PGSQL"=w355:refnum<class "LV-Data.PGSQL.lvclass">, "variable address"=w354:string, "data in"=w353:variant, "Time"=w349:timestamp)
            n119 = call "Write Or Not.vi"("Time"=w349, "data in"=w353) -> ("Write?"=w351:bool)  [unwired: 1 in]
            n120 = case shown="False" w351 {
              tunnel: [w367 w378] -> w361
              tunnel: [w370 w385] -> w360
              tunnel: w356 -> [w367 w384]
              tunnel: w355 -> [w370 w383]
              tunnel: w354 -> [_ w382]
              tunnel: [TRUE ("Wrote to DB?") w373] -> w350
              tunnel: w353 -> [_ w380]
              tunnel: [w369 w377] -> w352
              tunnel: w349 -> [w369 _]
              tunnel: ["Write Not Attempted" w372] -> w348
              tunnel: [w365 w371] -> w346
              frame False {
                n121 = Get Date/Time In Seconds() -> (seconds since 1Jan1904=w365:timestamp)
              }
              frame True {
                n122 = call "Shorten Cluster.vi"("error in (no error)"=w384, "Variant"=w380, "variable address in"=w382) -> ("error out"=w379:errorcluster, "Variant"=w376:variant, "variable address out"=w381:string)
                n123 = Get Date/Time In Seconds() -> (seconds since 1Jan1904=w377:timestamp)
                n124 = call-poly <userlib>:"Write Variable.vi"("error in (no error)"=w379, "Data"=w376, "variable"=w381, "Data.PG in"=w383) -> ("error out"=w378:errorcluster, "Wrote to DB?"=w373:bool, "Data.PG out"=w385:refnum<class "LV-Data.PGSQL.lvclass">)  [unwired: 4 in, 1 out]
                n125 = Select(t="Write Succesful", s=w373, f="Write Failed") -> (s? t:f=w372:string)
                n126 = Get Date/Time In Seconds() -> (seconds since 1Jan1904=w371:timestamp)
              }
            }
            n127 = Format Into String(w348, w346) -> (resulting string=w345:string)  [unwired: 3 in, 1 out]
            n128 = Bundle By Name(cluster=w359, "Data.PGSQL"=w360, "Time"=w352) -> (w358:T4)
            n129 = call <vilib>:"Build State String with Arguments__JKI_lib_State_Machine.vi"("Arguments (\"\")"=w345, "State"="UI: Update Status") -> ("State with Arguments"=w341:string)  [unwired: 4 in]
            n130 = Select(t="", s=w350, f="PGSQL: Close\nPGSQL: Open") -> (s? t:f=w344:string)
            n131 = call <vilib>:"Add State(s) to Queue__jki_lib_state_machine.vi"("State(s) in Front (\"\")"=w341, "State(s) at Back (\"\")"=w344) -> ("States Out"=w342:string)  [unwired: 13 in]
            n132 = call <vilib>:"Add State(s) to Queue__JKI_lib_State_Machine.vi"("State(s) in Front (\"\")"=w342, "State(s) in (\"\")"=w364) -> ("States Out"=w363:string)  [unwired: 13 in]
          }
          frame "PGSQL: Read" {
            n133 = Unbundle By Name(w387) -> ("SelfRef"=w390:refnum<class "Logger.PGSQL.lvclass">, "Data.PGSQL"=w389:refnum<class "LV-Data.PGSQL.lvclass">, "variable address"=w386:string)
            n134 = case shown="Default" w386 {
              selector: w386 -> [_ w396]
              tunnel: [w395 w402] -> w391
              tunnel: w390 -> [_ w401]
              tunnel: w389 -> [_ w398]
              tunnel: w388 -> [w395 w397]
              frame "" {
              }
              frame Default {
                n135 = call-poly <userlib>:"Read Variable.vi"("error in (no error)"=w397, "PG path"=w396, "Data.PGQL in"=w398) -> ("error out"=w399:errorcluster, "Value"=w400:string)  [unwired: 3 in, 4 out]
                n136 = call "Logger.ReadVariable.vi"("error in (no error)"=w399, "Data"=w400, "Address"=w396, "Logger"=w401) -> ("error out"=w402:errorcluster)  [unwired: 6 in, 1 out]
              }
            }
            n137 = call <vilib>:"Add State(s) to Queue__JKI_lib_State_Machine.vi"("State(s) in (\"\")"=w394) -> ("States Out"=w393:string)  [unwired: 14 in]
          }
          frame "PGSQL: Close" {
            n138 = Unbundle By Name(w406) -> ("Data.PGSQL"=w408:refnum<class "LV-Data.PGSQL.lvclass">)
            n139 = call-dynamic "Close.vi"("error in (no error)"=w404, "Data.PG in"=w408) -> ("error out"=w403:errorcluster, "Data.PG out"=w407:refnum<class "LV-Data.PGSQL.lvclass">)  [unwired: 8 in]
            n140 = Bundle By Name(cluster=w406, "Data.PGSQL"=w407) -> (w405:T4)
            n141 = call <vilib>:"Add State(s) to Queue__JKI_lib_State_Machine.vi"("State(s) in (\"\")"=w411) -> ("States Out"=w410:string)  [unwired: 14 in]
          }
        }
      }
    }
    frame Error {
    }
  }
  n142 = call-parent "Process.vi"("error in"=w5, "SMO"=w4) -> ("error out"=w3:errorcluster, "SMO out"=→"Logger out":refnum<class "Logger.PGSQL.lvclass">)  [unwired: 8 in]
  n143 = Merge Errors(w3, w2) -> (→"error out":errorcluster)
